vi "Sensor de presion_HEGO.vi"() -> ()   [LabVIEW 2015]
uses:
  <vilib>/MakerHub/LINX/Public/Peripherals/Analog/Analog Read 1 Chan.vi
  <vilib>/MakerHub/LINX/Public/Peripherals/Analog/Analog Read N Chans.vi
  <vilib>/MakerHub/LINX/Private/Local IO/LinxAnalogRead.vi
  <vilib>/MakerHub/LINX/Public/Utilities/Check Channel.vi
  <vilib>/MakerHub/LINX/Public/Utilities/Open Serial.vi
  <vilib>/MakerHub/LINX/Private/Utilties/Generate Error.vi
  <vilib>/MakerHub/LINX/LMH-LINX.lvlib
panel:
  in  "Analog Channel":u8
  in  "Serial Port":refnum<visa-resource-name>="N/A"
  out "?":string
  out "Waveform Chart":dbl(graph)
  out "Gauge":dbl(knob) scale=0.0..700.0
  in  "?":bool
  out "?":bool
  out "?":bool
  out "?":bool
  out "SENSOR DE VOLTAJE":dbl(knob) scale=0.0..5.0
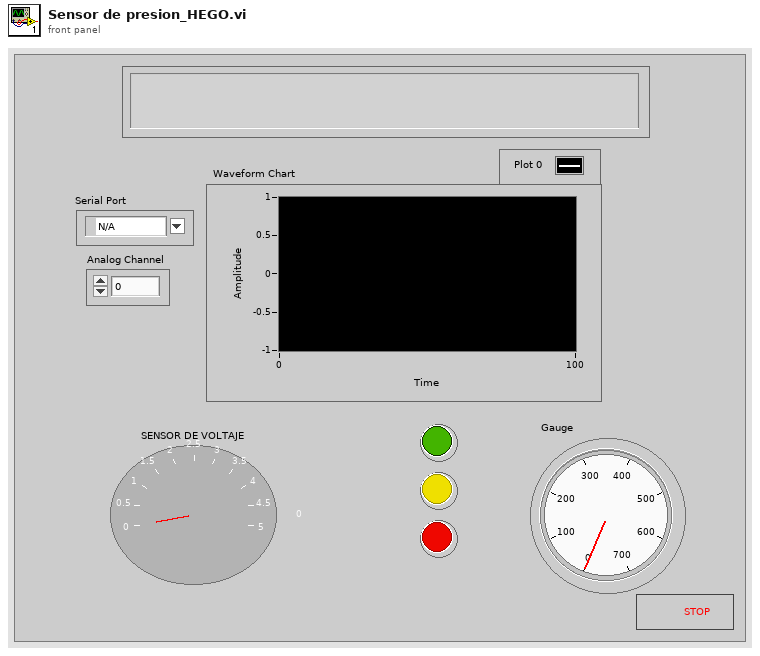
[diagram p1: front panel]
types:
  T1 = typedef "LMH-LINX.lvlib/LINX Ref.ctl" = cluster{"IO":T2, "Interface":T3, "LINX Device Config":T4}
  T2 = typedef "LMH-LINX.lvlib/Platform.ctl" = enum16{"Remote", "Local"}
  T3 = typedef "LMH-LINX.lvlib/Interface.ctl" = enum16{"Serial", "TCP"}
  T4 = typedef "LMH-LINX.lvlib/Device.lvlib/LINX Device Config.ctl" = cluster{"Interface":T3, "COM Port":refnum<visa-resource-name>, "TCP Configuration":T5, "Device Family":u8, "Device ID":u8, "Device Name":string, "TCP Ref":refnum<k5>, "Channels":T6}
  T5 = typedef "LMH-LINX.lvlib/Device.lvlib/TCP Config.ctl" = cluster{"IP Address":string, "Port":u16}
  T6 = typedef "LMH-LINX.lvlib/Channels.ctl" = cluster{"DI":u8[], "DO":u8[], "AI":u8[], "AO":u8[], "PWM":u8[], "QE":u8[], "UART":u8[], "I2C 2":u8[], "SPI":u8[], "CAN":u8[], "Servo":u8[], "AI Ref (V)":dbl, "AI Resolution (Bits)":u8, "AO Ref (V)":dbl, "AO Resolution (Bits)":u8}
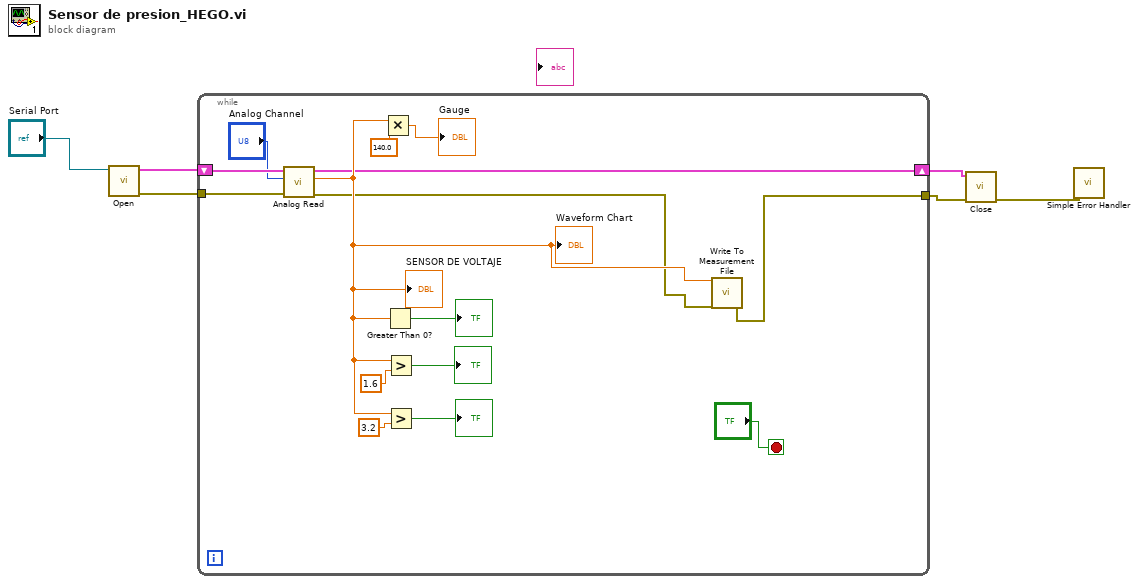
[diagram p0: block diagram]
diagram:
  n1 = call-poly <vilib>:"Open.vi"("Serial Port"="Serial Port") -> ("Error Out"=w4:errorcluster, "LINX Resource"=w5:T1)  [unwired: 8 in, 1 out]
  n2 = while {
    tunnel: [w13] -> w6
    shift-right: [w10] -> w3
    shift-left: w5 -> [w9]
    tunnel: w4 -> [w8]
    stop <- "?" stop-if-true
    n3 = call-poly <vilib>:"Analog Read.vi"("Error In"=w8, "Analog Channel"="Analog Channel", "LINX Resource"=w9) -> ("Error Out"=w11:errorcluster, "Voltage"=w12:dbl, "LINX Resource"=w10:T1)  [unwired: 5 in, 1 out]
    "SENSOR DE VOLTAJE" <- w12
    "Waveform Chart" <- w12
    n4 = Multiply(x=w12, y=140.0) -> (x*y=→"Gauge":dbl)
    n5 = Greater Than 0?(x=w12) -> (x > 0?=→"?":bool)
    n6 = Greater?(x=w12, y=1.6) -> (0:→"?":bool)
    n7 = Greater?(x=w12, y=3.2) -> (0:→"?":bool)
    n8 = call "Write To Measurement File"("Signals"=w12, "error in (no error)"=w11) -> ("error out"=w13:errorcluster)  [unwired: 15 in, 2 out]
  }
  n9 = call <vilib>:"Close.vi"("Error In"=w6, "LINX Resource"=w3) -> ("Error Out"=w2:errorcluster)  [unwired: 9 in]
  n10 = call <vilib>:"Simple Error Handler.vi"("error in (no error)"=w2) -> ()  [unwired: 4 in, 5 out]
